vi "Main.vi"(8 "error in":errorcluster, 11 "Abstract Hardware in":refnum<class "Abstract Hardware.lvclass">) -> (0 "error out":errorcluster, 3 "Abstract Hardware out":refnum<class "Abstract Hardware.lvclass">)   [LabVIEW 2020, in "Abstract Hardware.lvclass"]
doc: "The <b>Queued Message Handler</b> of the Worker that owns this VI."
uses:
  Abstract Hardware.lvclass
  C:/Program Files (x86)/National Instruments/LabVIEW 2020/vi.lib/addons/_Workers/Library/Classes/Worker/Worker.lvclass
  Initialization Data.ctl
  Response Cases.ctl
  Abstract Hardware.lvclass/Abstract Hardware.ctl
  <vilib>/addons/_Workers/Library/Classes/Message Queue/Message Queue.lvclass
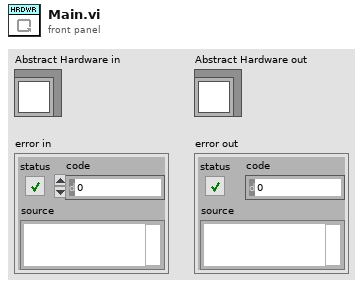
[diagram p1: front panel]
types:
  T1 = typedef "Abstract Hardware.lvclass/Initialization Data.ctl" = cluster{"Response Cases":T2}
  T2 = typedef "Abstract Hardware.lvclass/Response Cases.ctl" = cluster{"Placeholder - Can be deleted":string}
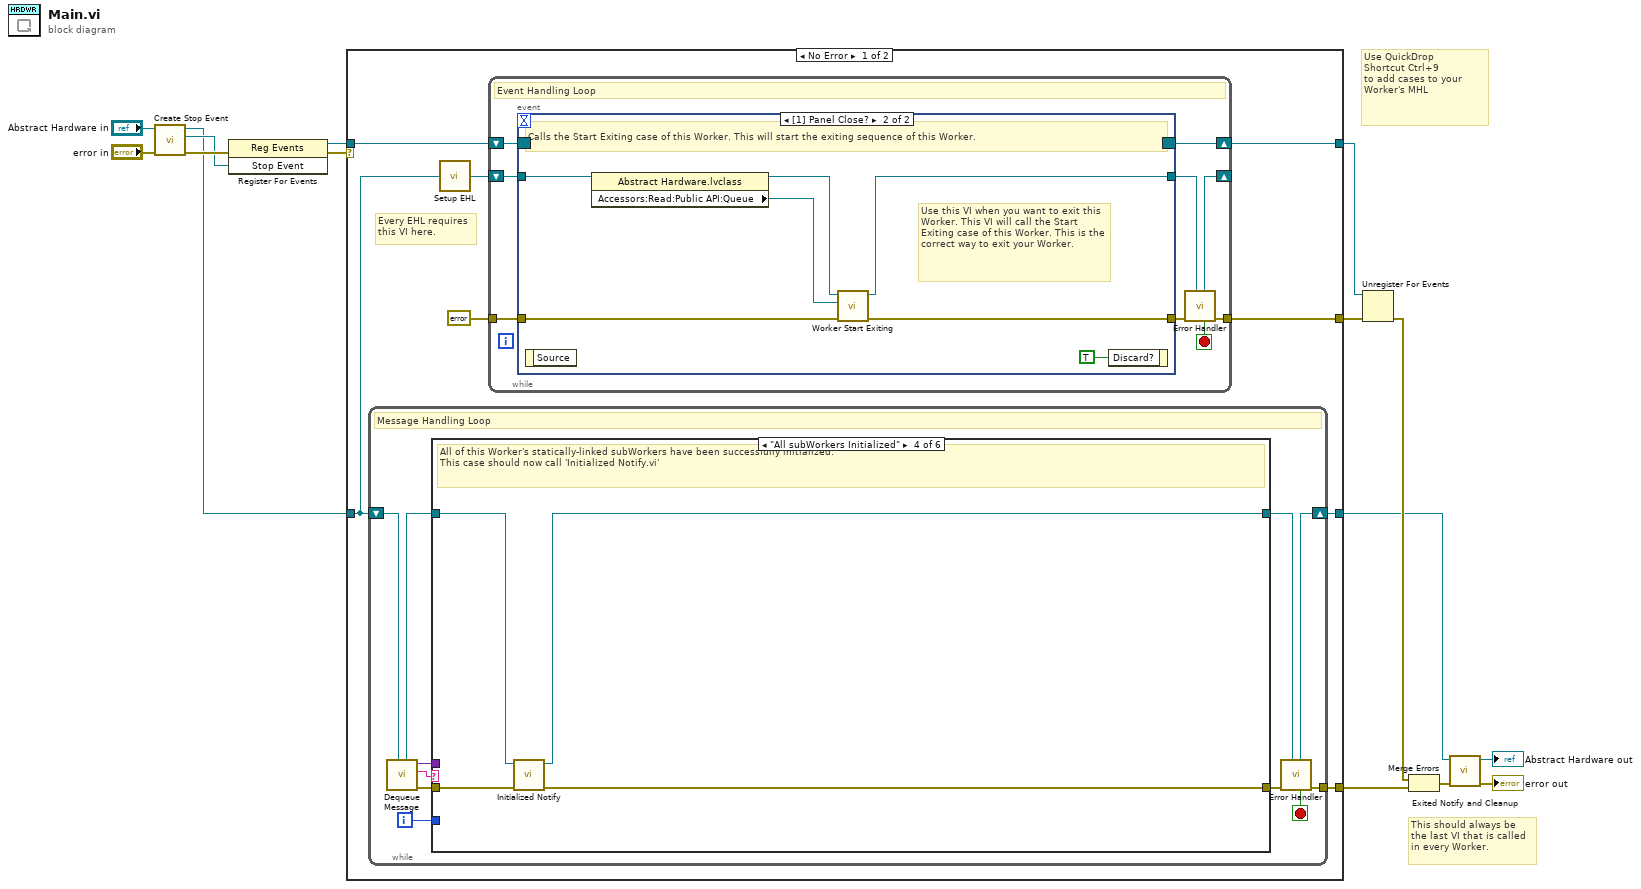
[diagram p0: block diagram]
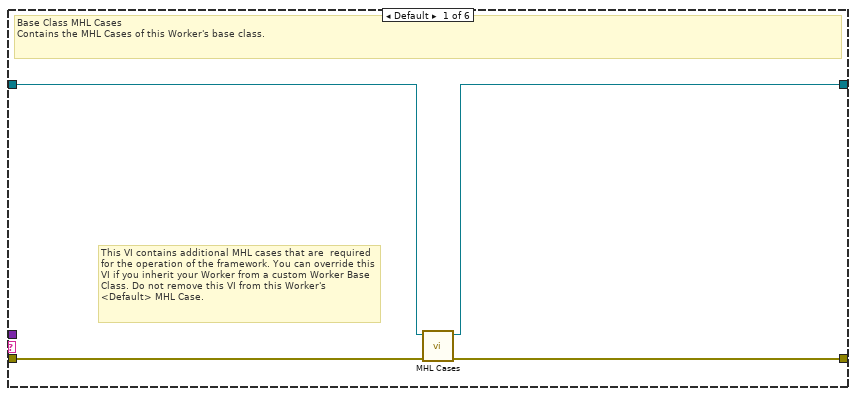
[diagram p2: hidden frame]
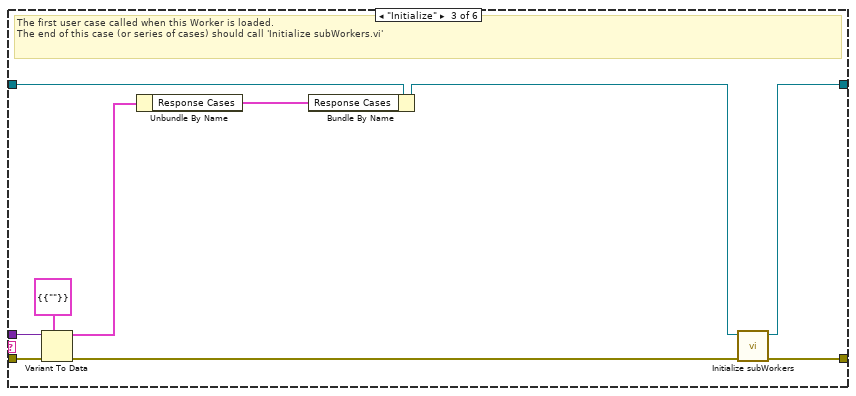
[diagram p4: hidden frame]
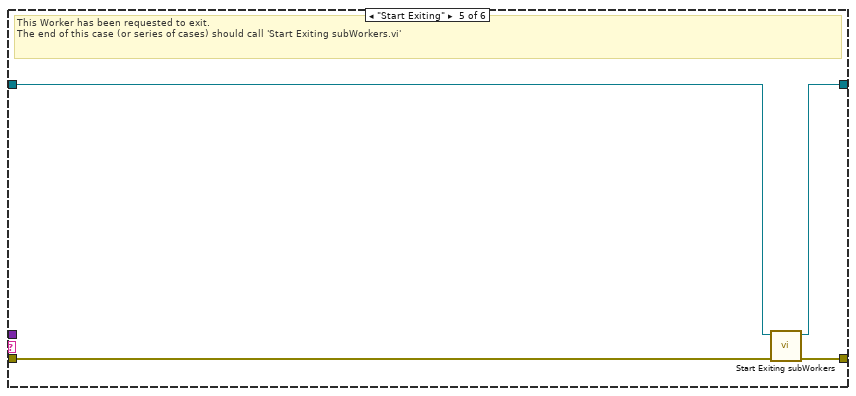
[diagram p5: hidden frame]
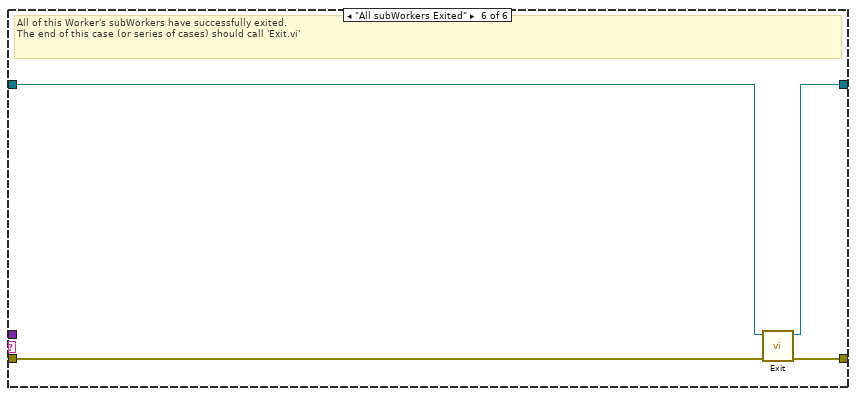
[diagram p6: hidden frame]
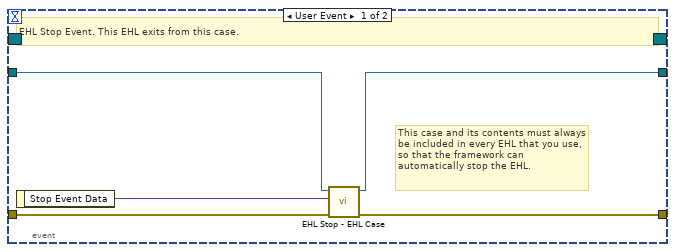
[diagram p7: hidden frame]
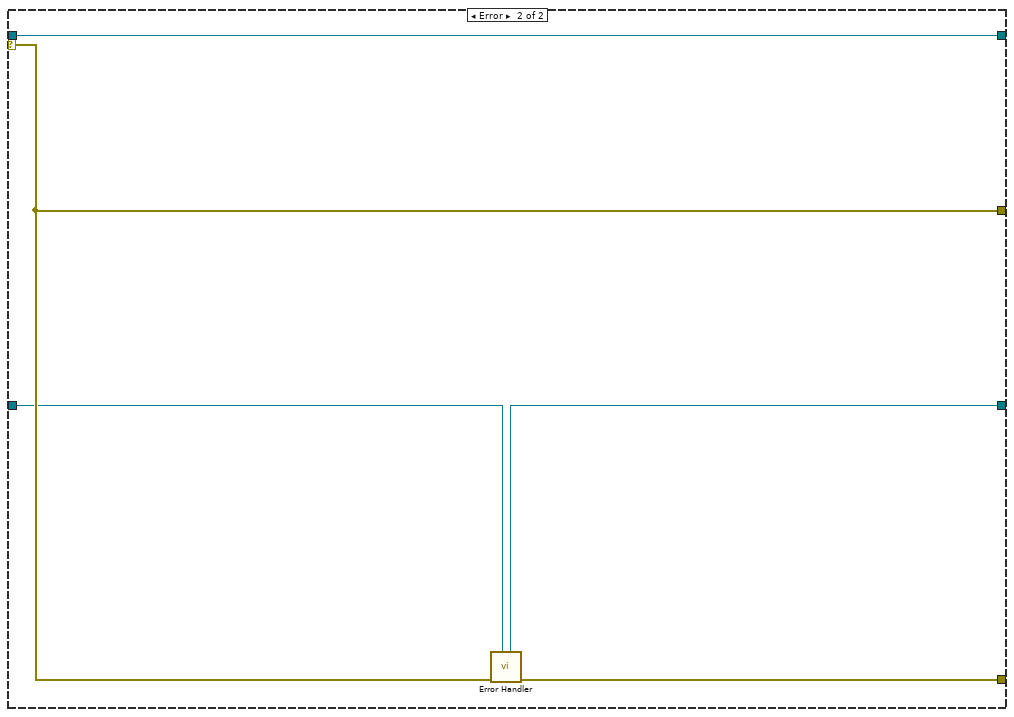
[diagram p8: hidden frame]
diagram:
  # "Use QuickDrop\nShortcut Ctrl+9\nto add cases to your\nWorker's MHL"
  # "This should always be the last VI that is called in every Worker."
  n1 = call-dynamic "Create Stop Event.vi"("error in"="error in", "Worker"="Abstract Hardware in") -> ("error out"=w10:errorcluster, "Stop Event"=w7:refnum<user-event>, "Worker out"=w4:refnum<class "Abstract Hardware.lvclass">)  [unwired: 7 in]
  n2 = register-events(error in=w10, w7) -> (reference out=w9:refnum<event-registration>, error out=w1:errorcluster)  [unwired: 1 in]
  n3 = case shown="No Error" w1 {
    tunnel: w4 -> [w18 w85]
    tunnel: [w16 w86] -> w8
    tunnel: w9 -> [w23 w87]
    tunnel: [w20 w88] -> w14
    tunnel: [w22 w87] -> w13
    tunnel: [w17 w84] -> w11
    selector: w1 -> [_ w88]
    frame No Error {
      # "Every EHL requires\nthis VI here."
      n4 = while {
        shift-right: [w32] -> w17
        shift-left: w18 -> [w34]
        tunnel: [w33] -> w16
        i -> [w24]
        stop <- w25 stop-if-true
        # "Message Handling Loop"
        n5 = call-dynamic "Dequeue Message.vi"("Worker"=w34) -> ("error out"=w31:errorcluster, "Case out"=w26:string, "Data out"=w27:variant, "Worker out"=w29:refnum<class "Abstract Hardware.lvclass">)  [unwired: 6 in, 1 out]
        n6 = case "Worker MHL Case Structure (DO NOT CHANGE LABEL NAME)" shown="\"All subWorkers Initialized\"" w26 {
          tunnel: w31 -> [w38 w39 w48 w52 w55 w62]
          tunnel: [w37 w39 w50 w51 w58 w61] -> w30
          tunnel: w29 -> [w36 w40 w47 w54 w56 w60]
          tunnel: [w35 w40 w49 w53 w57 w59] -> w28
          tunnel: w27 -> [_ _ w45 _ _ _]
          tunnel: w24 -> [_ _ _ _ _ _]
          frame Default {
            # "This VI contains additional MHL cases that are  required for the operation of the framework. You can override this VI if you inherit your Worker from a custom Worker Base Class. Do not remove this VI from this Worker's <Default> MHL Case."
            # "Base Class MHL Cases\nContains the MHL Cases of this Worker's base class."
            n7 = call-dynamic "MHL Cases.vi"("error in"=w38, "Worker in"=w36) -> ("error out"=w37:errorcluster, "Worker out"=w35:refnum<class "Abstract Hardware.lvclass">)  [unwired: 8 in]
          }
          frame "------------ FRAMEWORK CASES -----------" {
            # "Start of Workers Framework Cases"
          }
          frame "Initialize" {
            # "The first user case called when this Worker is loaded.\nThe end of this case (or series of cases) should call 'Initialize subWorkers.vi'"
            n8 = Variant To Data(error in=w48, type=T1 {"Response Cases"={"Placeholder - Can be deleted"=""}} ("Initialization Data"), Variant=w45) -> (data=w43:T1, error out=w46:errorcluster)
            n9 = Unbundle By Name(w43) -> ("Response Cases"=w42:T2)
            n10 = Bundle By Name(cluster=w47, "Response Cases"=w42) -> (w44:refnum<class "Abstract Hardware.lvclass">)
            n11 = call-dynamic "Initialize subWorkers.vi"("error in"=w46, "Worker"=w44) -> ("error out"=w50:errorcluster, "dup Worker out"=w49:refnum<class "Abstract Hardware.lvclass">)  [unwired: 8 in]
          }
          frame "All subWorkers Initialized" {
            # "All of this Worker's statically-linked subWorkers have been successfully initialized.\nThis case should now call 'Initialized Notify.vi'"
            n12 = call-dynamic "Initialized Notify.vi"("error in"=w52, "Worker"=w54) -> ("error out"=w51:errorcluster, "dup Worker out"=w53:refnum<class "Abstract Hardware.lvclass">)  [unwired: 8 in]
          }
          frame "Start Exiting" {
            # "This Worker has been requested to exit. \nThe end of this case (or series of cases) should call 'Start Exiting subWorkers.vi'"
            n13 = call-dynamic "Start Exiting subWorkers.vi"("error_in"=w55, "Worker"=w56) -> ("error out"=w58:errorcluster, "dup Worker out"=w57:refnum<class "Abstract Hardware.lvclass">)  [unwired: 8 in]
          }
          frame "All subWorkers Exited" {
            # "All of this Worker's subWorkers have successfully exited. \nThe end of this case (or series of cases) should call 'Exit.vi'"
            n14 = call-dynamic "Exit.vi"("error_in"=w62, "Worker"=w60) -> ("error out"=w61:errorcluster, "dup Worker out"=w59:refnum<class "Abstract Hardware.lvclass">)  [unwired: 8 in]
          }
        }
        n15 = call-dynamic "Error Handler.vi"("Worker"=w28, "error_in"=w30) -> ("error out"=w33:errorcluster, "Stop Loop"=w25:bool, "Worker out"=w32:refnum<class "Abstract Hardware.lvclass">)  [unwired: 7 in]
      }
      n16 = call-dynamic "Setup EHL.vi"("Worker"=w18) -> ("Worker out"=w19:refnum<class "Abstract Hardware.lvclass">)  [unwired: 14 in]
      n17 = while "Event Handling Loop" {
        shift-right: [w71] -> w22
        shift-left: w23 -> [w70]
        tunnel: [w66] -> w20
        tunnel: errorcluster {"status"=FALSE, "code"=0, "source"=""} ("error constant") -> [w68]
        shift-right: [w64] -> _
        shift-left: w19 -> [w69]
        stop <- w63 stop-if-true
        # "Event Handling Loop"
        n18 = event shown="[1] Panel Close?" {
          selector: w70 -> [_ _]
          dyn-events: [_ _] -> w71
          timeout: _ -> [_ _]
          tunnel: [w75 w82] -> w67
          tunnel: w68 -> [w76 w81]
          tunnel: w69 -> [w74 w80]
          tunnel: [w73 w79] -> w65
          event User Event {
            # "This case and its contents must always be included in every EHL that you use, so that the framework can automatically stop the EHL."
            # "EHL Stop Event. This EHL exits from this case."
            n19 = event-data() -> ("Stop Event Data"=w72:variant)  [unwired: 1 in]
            n20 = call-dynamic "EHL Stop - EHL Case.vi"("error in"=w76, "Stop Event Data"=w72, "Worker"=w74) -> ("error out"=w75:errorcluster, "Worker out"=w73:refnum<class "Abstract Hardware.lvclass">)  [unwired: 7 in]
          }
          event Panel Close? {
            # "Use this VI when you want to exit this Worker. This VI will call the Start Exiting case of this Worker. This is the correct way to exit your Worker."
            # "Calls the Start Exiting case of this Worker. This will start the exiting sequence of this Worker."
            n21 = event-data() -> ()  [unwired: 1 in, 1 out]
            n22 = property class="Abstract Hardware.lvclass"(reference=w80) -> (reference out=w78:refnum<class "Abstract Hardware.lvclass">, "Accessors:Read:Public API:Queue"=w77:refnum<class "Message Queue.lvclass">)  [unwired: 1 in, 1 out]
            n23 = call-dynamic "Worker Start Exiting.vi"("error_in"=w81, "Message Queue"=w77, "Worker"=w78) -> ("error out"=w82:errorcluster, "dup Worker out"=w79:refnum<class "Abstract Hardware.lvclass">)  [unwired: 7 in]
            n24 = event-data("Discard?"=TRUE) -> ()  [unwired: 1 in, 1 out]
          }
        }
        n25 = call-dynamic "Error Handler.vi"("Worker"=w65, "error_in"=w67) -> ("error out"=w66:errorcluster, "Stop Loop"=w63:bool, "Worker out"=w64:refnum<class "Abstract Hardware.lvclass">)  [unwired: 7 in]
      }
    }
    frame Error {
      n26 = call-dynamic "Error Handler.vi"("Worker"=w85, "error_in"=w88) -> ("error out"=w86:errorcluster, "Worker out"=w84:refnum<class "Abstract Hardware.lvclass">)  [unwired: 7 in, 1 out]
    }
  }
  n27 = Unregister For Events(event registration refnum=w13, error in=w14) -> (error out=w15:errorcluster)
  n28 = Merge Errors(w15, w8) -> (w12:errorcluster)
  n29 = call-dynamic "Exited Notify and Cleanup.vi"("error_in"=w12, "Worker"=w11) -> ("error out"=→"error out":errorcluster, "dup Worker out"=→"Abstract Hardware out":refnum<class "Abstract Hardware.lvclass">)  [unwired: 8 in]
